vi "Z900_navX_SERIAL_CapturePacket.vi"(11 "Buffer":string) -> (0 "Packet Size":i32, 1 "Packet Located":bool, 2 "Packet":string, 3 "Buffer":string)   [LabVIEW 2017, in "navX Library v2.lvlib"]
uses:
  navX Library v2.lvlib
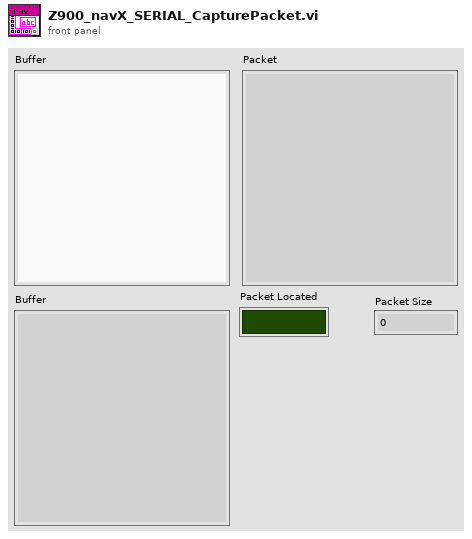
[diagram p1: front panel]
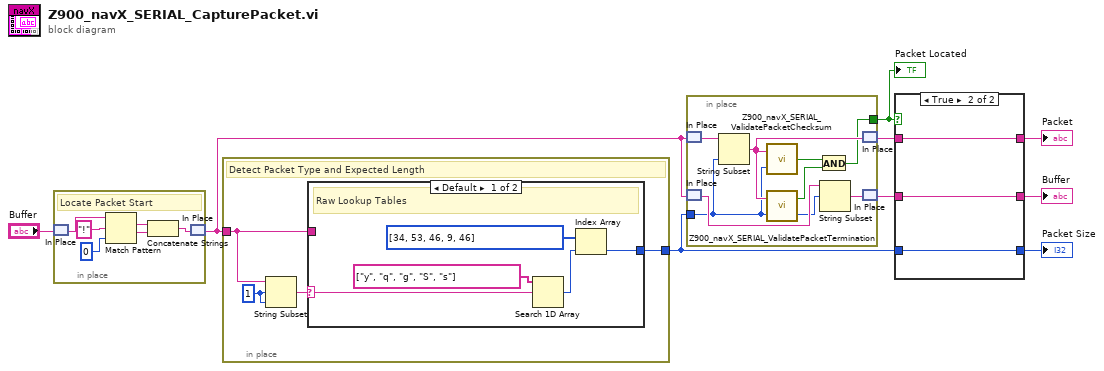
[diagram p0: block diagram]
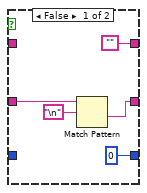
[diagram p2: hidden frame]
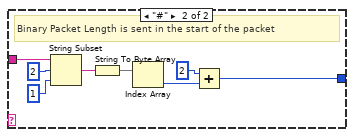
[diagram p3: hidden frame]
diagram:
  n1 = in-place {
    # "Locate Packet Start"
    n2 = in-place-match #1("Buffer") -> (w12:string)
    n3 = Match Pattern(string=w12, regular expression="!" ("Packet Start Char"), offset (0)=0 ("offset past match")) -> (match substring=w15:string, after substring=w14:string)  [unwired: 2 out]
    n4 = Concatenate Strings(w15, w14) -> (w11:string)
    n5 = in-place-match #1(w11) -> (w8:string)
  }
  n6 = in-place {
    in-place-border: w8 -> [w17]
    in-place-border: [w16] -> w1
    w19 = 1 ("length (rest)")
    # "Detect Packet Type and Expected Length"
    n7 = String Subset(string=w17, offset (0)=w19, length (rest)=w19) -> (substring=w18:string)
    n8 = case shown="Default" w18 {
      selector: w18 -> [w20 _]
      tunnel: [w21 w28] -> w16
      tunnel: w17 -> [_ w26]
      frame Default {
        # "Raw Lookup Tables"
        n9 = Search 1D Array(1D array=string[] ["y", "q", "g", "S", "s"], element=w20) -> (index of element=w22:i32)  [unwired: 1 in]
        n10 = Index Array(array=i32[] [34, 53, 46, 9, 46], index=w22) -> (element=w21:i32)
      }
      frame "#" {
        # "Binary Packet Length is sent in the start of the packet"
        n11 = String Subset(string=w26, offset (0)=2, length (rest)=1 ("length (rest)")) -> (substring=w27:string)
        n12 = String To Byte Array(string=w27) -> (unsigned byte array=w30:u8[])
        n13 = Index Array(array=w30) -> (element=w31:u8)  [unwired: 1 in]
        n14 = Add(x=u8 2 ("y"), y=w31) -> (x+y=w28:u8)
      }
    }
  }
  n15 = in-place {
    in-place-border: w1 -> [w37]
    in-place-border: [w34] -> w7
    n16 = in-place-match #2(w8) -> (w39:string)
    n17 = in-place-match #3(w8) -> (w40:string)
    n18 = String Subset(string=w39, length (rest)=w37) -> (substring=w38:string)  [unwired: 1 in]
    n19 = call "Z900_navX_SERIAL_ValidatePacketChecksum.vi"("Expected Packet Length"=w37, "Buffer"=w38) -> ("Packet Valid"=w36:bool)
    n20 = call "Z900_navX_SERIAL_ValidatePacketTermination.vi"("Expected Packet Length"=w37, "Buffer"=w38) -> ("Packet Termination Offset"=w33:i32, "Packet Valid"=w35:bool)
    n21 = And(x=w36, y=w35) -> (x .and. y?=w34:bool)
    n22 = String Subset(string=w40, offset (0)=w33) -> (substring=w41:string)  [unwired: 1 in]
    n23 = in-place-match #2(w38) -> (w5:string)
    n24 = in-place-match #3(w41) -> (w3:string)
  }
  "Packet Located" <- w7
  n25 = case shown="True" w7 {
    tunnel: ["" w49] -> w6
    tunnel: w5 -> [_ w49]
    tunnel: [w43 w48] -> w4
    tunnel: w3 -> [w45 w48]
    tunnel: [0 w47] -> w2
    tunnel: w1 -> [_ w47]
    frame False {
      n26 = Match Pattern(string=w45, regular expression="\n") -> (after substring=w43:string)  [unwired: 1 in, 3 out]
    }
    frame True {
    }
  }
  "Packet" <- w6
  "Buffer" <- w4
  "Packet Size" <- w2
